vi "PC Main.vi"() -> ()   [LabVIEW 2021]
panel:
  in  "stop":bool
  out "Button0":bool
  out "LED3":bool
  out "LED2":bool
  out "LED1":bool
  out "LED0":bool
  out "Pause Led2i":bool
  out "Led1i":bool
  out "Led0i":bool
  out "Led3i":bool
  in  "Count(mSec)":u32
  in  "Pause":bool
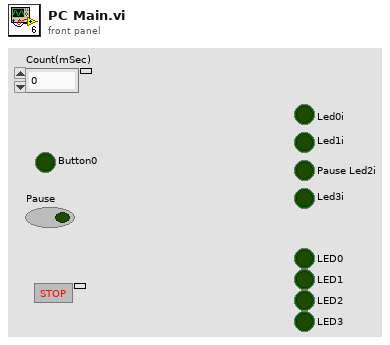
[diagram p1: front panel]
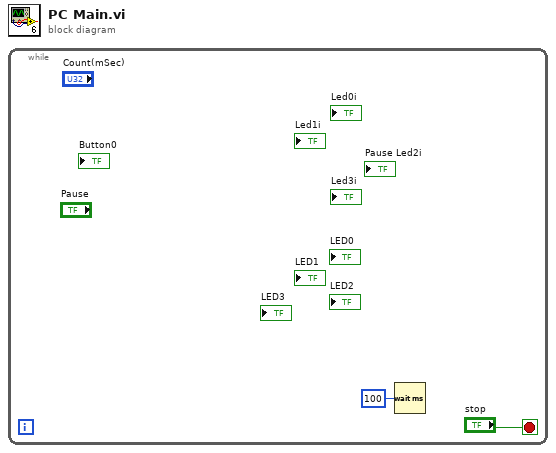
[diagram p0: block diagram]
diagram:
  n1 = while {
    stop <- "stop" stop-if-true
    n2 = Wait (ms)(milliseconds to wait=u32 100) -> ()  [unwired: 1 out]
  }
